vi "pho_DB_Insert_LIV_meas_recipe.vi"(0 "V start":dbl=-1.0, 1 "Sweep Direction (Keysight)":i32(ring) items=["Up", "Down"], 5 "V end":dbl=0.4, 7 "points":u16=40, 9 "I compliance sweep":dbl=0.001, 11 "error in (no error)":errorcluster, 12 "sweep delay ms":dbl=500.0) -> (4 "RecipeID":string)   [LabVIEW 2012]
panel:
  out "Data":string[][](array[string])
  out "error out":errorcluster
  in  "DSN":string="DSN=pho_test"
  out "sql string":string
  # "Sweep Settings"
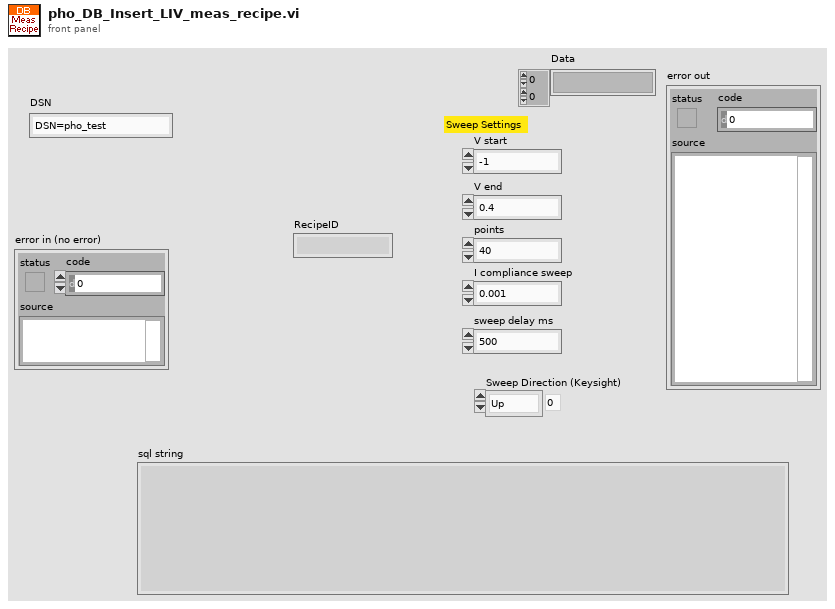
[diagram p1: front panel]
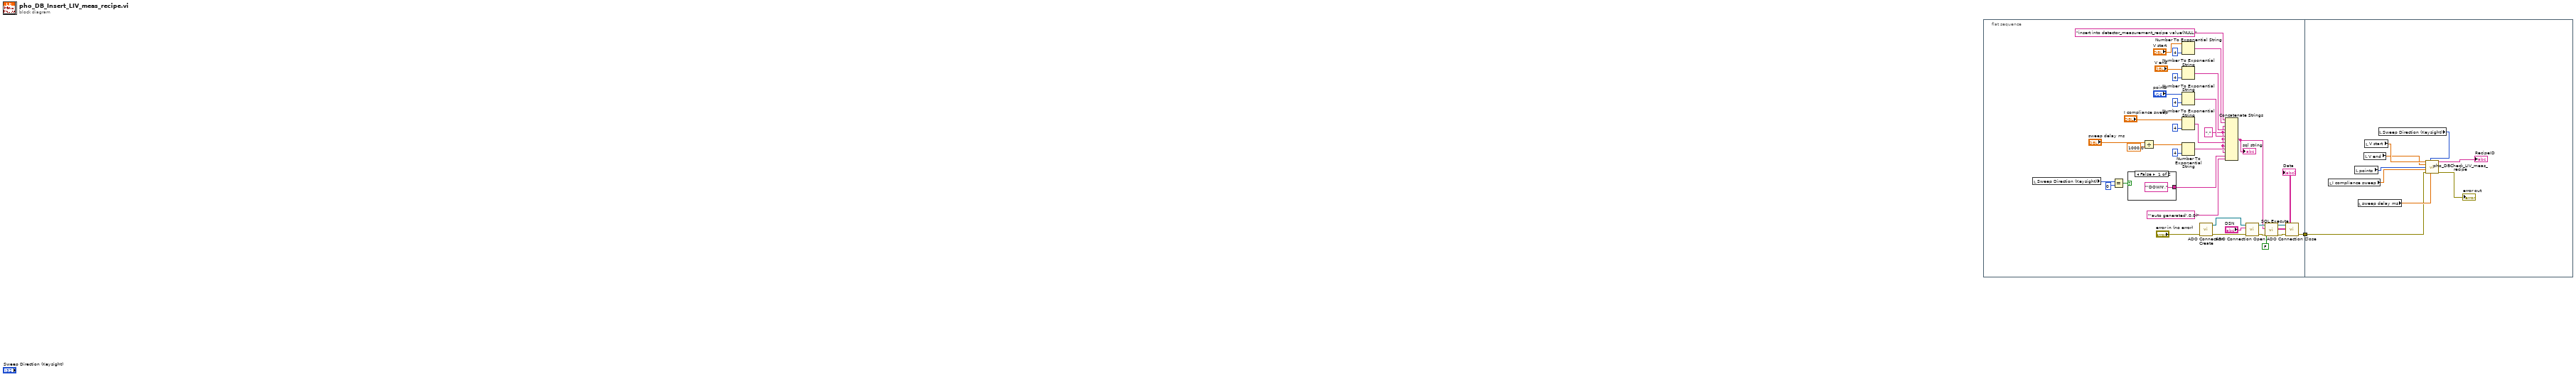
[diagram p0: block diagram]
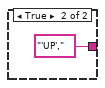
[diagram p2: hidden frame]
diagram:
  n1 = flat-sequence {
    tunnel: [w37] -> w1
    tunnel: w1 -> [w42]
    frame #0 {
      w9 = "," ("string")
      n2 = local read "Sweep Direction (Keysight)"() -> (w12:i32)
      n3 = Equal?(x=w12, y=0) -> (x = y?=w10:bool)
      n4 = case shown="False" w10 {
        tunnel: ["'DOWN'," ("string") "'UP'," ("string")] -> w8
        frame False {
        }
        frame True {
        }
      }
      n5 = Divide(x="sweep delay ms", y=1000.0) -> (x/y=w14:dbl)
      n6 = Number To Exponential String(number="V start", precision (6)=i16 4) -> (E-format string=w27:string)  [unwired: 2 in]
      n7 = Number To Exponential String(number="V end", precision (6)=i16 4) -> (E-format string=w24:string)  [unwired: 2 in]
      n8 = Number To Exponential String(number="points", precision (6)=i16 4) -> (E-format string=w21:string)  [unwired: 2 in]
      n9 = Number To Exponential String(number="I compliance sweep", precision (6)=i16 4) -> (E-format string=w18:string)  [unwired: 2 in]
      n10 = Number To Exponential String(number=w14, precision (6)=i16 4) -> (E-format string=w13:string)  [unwired: 2 in]
      n11 = call "ADO Connection Create.vi"("error in (no error)"="error in (no error)") -> ("error out"=w34:errorcluster, "ADODB._Connection Out"=w35:refnum<k7>)  [unwired: 9 in]
      n12 = Concatenate Strings("insert into detector_measurement_recipe value(NULL,", w27, w9, w24, w9, w21, w9, w18, w9, w13, w9, w8, "'auto generated',0,0)" ("string")) -> (w3:string)
      "sql string" <- w3
      n13 = call "ADO Connection Open.vi"("error in (no error)"=w34, "ConnectionString"="DSN", "ADODB._Connection In"=w35) -> ("error out"=w32:errorcluster, "ADODB._Connection Out"=w33:refnum<k7>)  [unwired: 7 in]
      n14 = call "SQL Execute.vi"("error in (no error)"=w32, "Return Data (T)"=FALSE, "Command Text"=w3, "ADODB._Connection In"=w33) -> ("error out"=w6:errorcluster, "Data"=→"Data":string[][], "ADODB._Connection Out"=w5:refnum<k7>)  [unwired: 4 in, 1 out]
      n15 = call "ADO Connection Close.vi"("error in (no error)"=w6, "ADODB._Connection In"=w5) -> ("error out"=w37:errorcluster)  [unwired: 8 in, 1 out]
    }
    frame #1 {
      n16 = local read "I compliance sweep"() -> (w45:dbl)
      n17 = local read "points"() -> (w46:u16)
      n18 = local read "sweep delay ms"() -> (w43:dbl)
      n19 = local read "V end"() -> (w47:dbl)
      n20 = local read "V start"() -> (w48:dbl)
      n21 = local read "Sweep Direction (Keysight)"() -> (w44:i32)
      n22 = call "pho_DBCheck_LIV_meas_recipe.vi"("V start"=w48, "Sweep Direction (Keysight)"=w44, "V end"=w47, "points"=w46, "I compliance sweep"=w45, "error in (no error)"=w42, "sweep delay ms"=w43) -> ("RecipeID"=→"RecipeID":string, "error out"=→"error out":errorcluster)  [unwired: 7 in]
    }
  }
